vi "Write Diff.vi"(0 "Device ID":T4(ring), 2 "Output_Direction":enum8{"Off", "Counter Clockwise", "Clockwise"}(ring), 5 "Module":T3(ring), 7 "Diff_Output":T2(ring), 9 "Output_PWM":T1(ring), 11 "error in":errorcluster) -> (4 "Device ID Out":T4(ring), 15 "error out":errorcluster)   [LabVIEW 2010]
doc: "This VI writes a single differential-ended digital PWM output signal to the transfer area."
uses:
  Robo Interface.dll
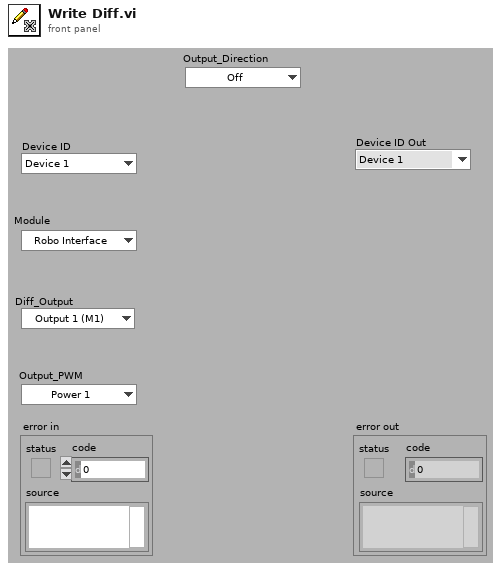
[diagram p1: front panel]
types:
  T1 = enum8{"Power 1", "Power 2", "Power 3", "Power 4", "Power 5", "Power 6", "Power 7", "Power 8"}
  T2 = enum8{"Output 1 (M1)", "Output 2 (M2)", "Output 3 (M3)", "Output 4 (M4)"}
  T3 = enum8{"Robo Interface", "Extension 1", "Extension 2", "Extension 3"}
  T4 = enum16{"Device 1", "Device 2", "Device 3", "Device 4", "Device 5", "Device 6", "Device 7", "Device 8"}
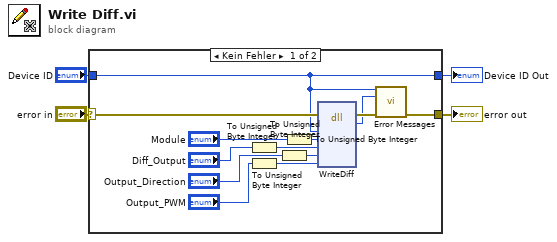
[diagram p0: block diagram]
diagram:
  n1 = case shown="Kein Fehler" "error in" {
    selector: "error in" -> [w17 w19]
    tunnel: [w11 w19] -> w1
    tunnel: "Device ID" -> [w5 w18]
    tunnel: [w5 w18] -> w2
    frame No Error {
      n2 = To Unsigned Byte Integer(number="Diff_Output") -> (unsigned 8bit integer=w8:u8)
      n3 = To Unsigned Byte Integer(number="Output_PWM") -> (unsigned 8bit integer=w10:u8)
      n4 = To Unsigned Byte Integer(number="Output_Direction") -> (unsigned 8bit integer=w9:u8)
      n5 = To Unsigned Byte Integer(number="Module") -> (unsigned 8bit integer=w7:u8)
      n6 = dll-call lib="D:/Aron/LabVIEW-Programmierung/a.F.b.u.s.A/robo_interface_distribute/Robo Interface/Advanced/Robo Interface.dll" fn="WriteDiff"(error in=w17, "Device_ID"=w5, "Module"=w7, "Diff_Output"=w8, "Output_Direction"=w9, "Output_PWM"=w10) -> (error out=w12:errorcluster, "return type"=w6:i32)  [unwired: 6 in, 2 out]
      n7 = call "Error Messages.vi"("Device ID"=w5, "Error Code"=w6, "error in (no error)"=w12) -> ("error out"=w11:errorcluster)  [unwired: 12 out]
    }
    frame Error {
    }
  }
  "error out" <- w1
  "Device ID Out" <- w2
